vi "界面1-项目.vi"() -> ()   [LabVIEW 2013]
uses:
  GlobleVar/IndentLevel.vi
panel:
  out "Boolean":bool
  in  "<-硬件配置":bool
  in  "试验->":bool
  in  "实验结果汇总":string(tree)
  in  "项目管理":string(tree)
  in  "分析数据":bool
  in  "打印报告":bool
  in  "新建":bool
  in  "删除":bool
  in  "刷新":bool
  in  "重命名":bool
  in  "还原":bool
  in  "新建油动机":bool
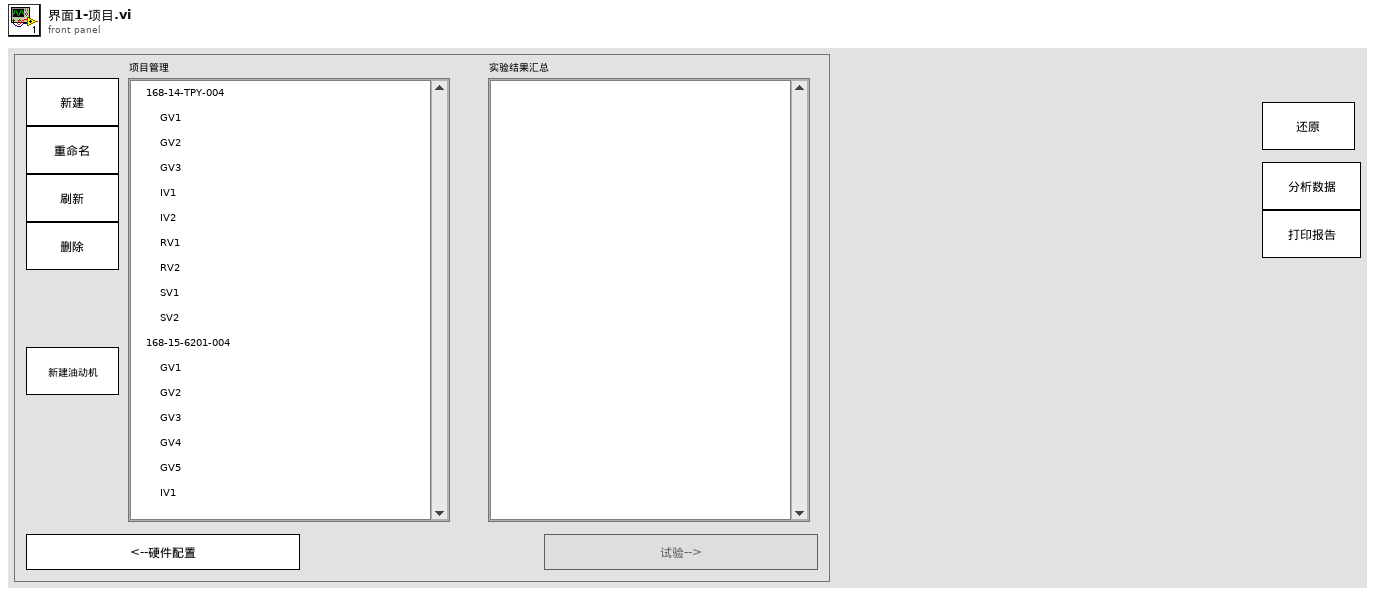
[diagram p1: front panel]
types:
  T1 = enum8{"Enabled", "Disabled", "Disabled and Grayed Out"}
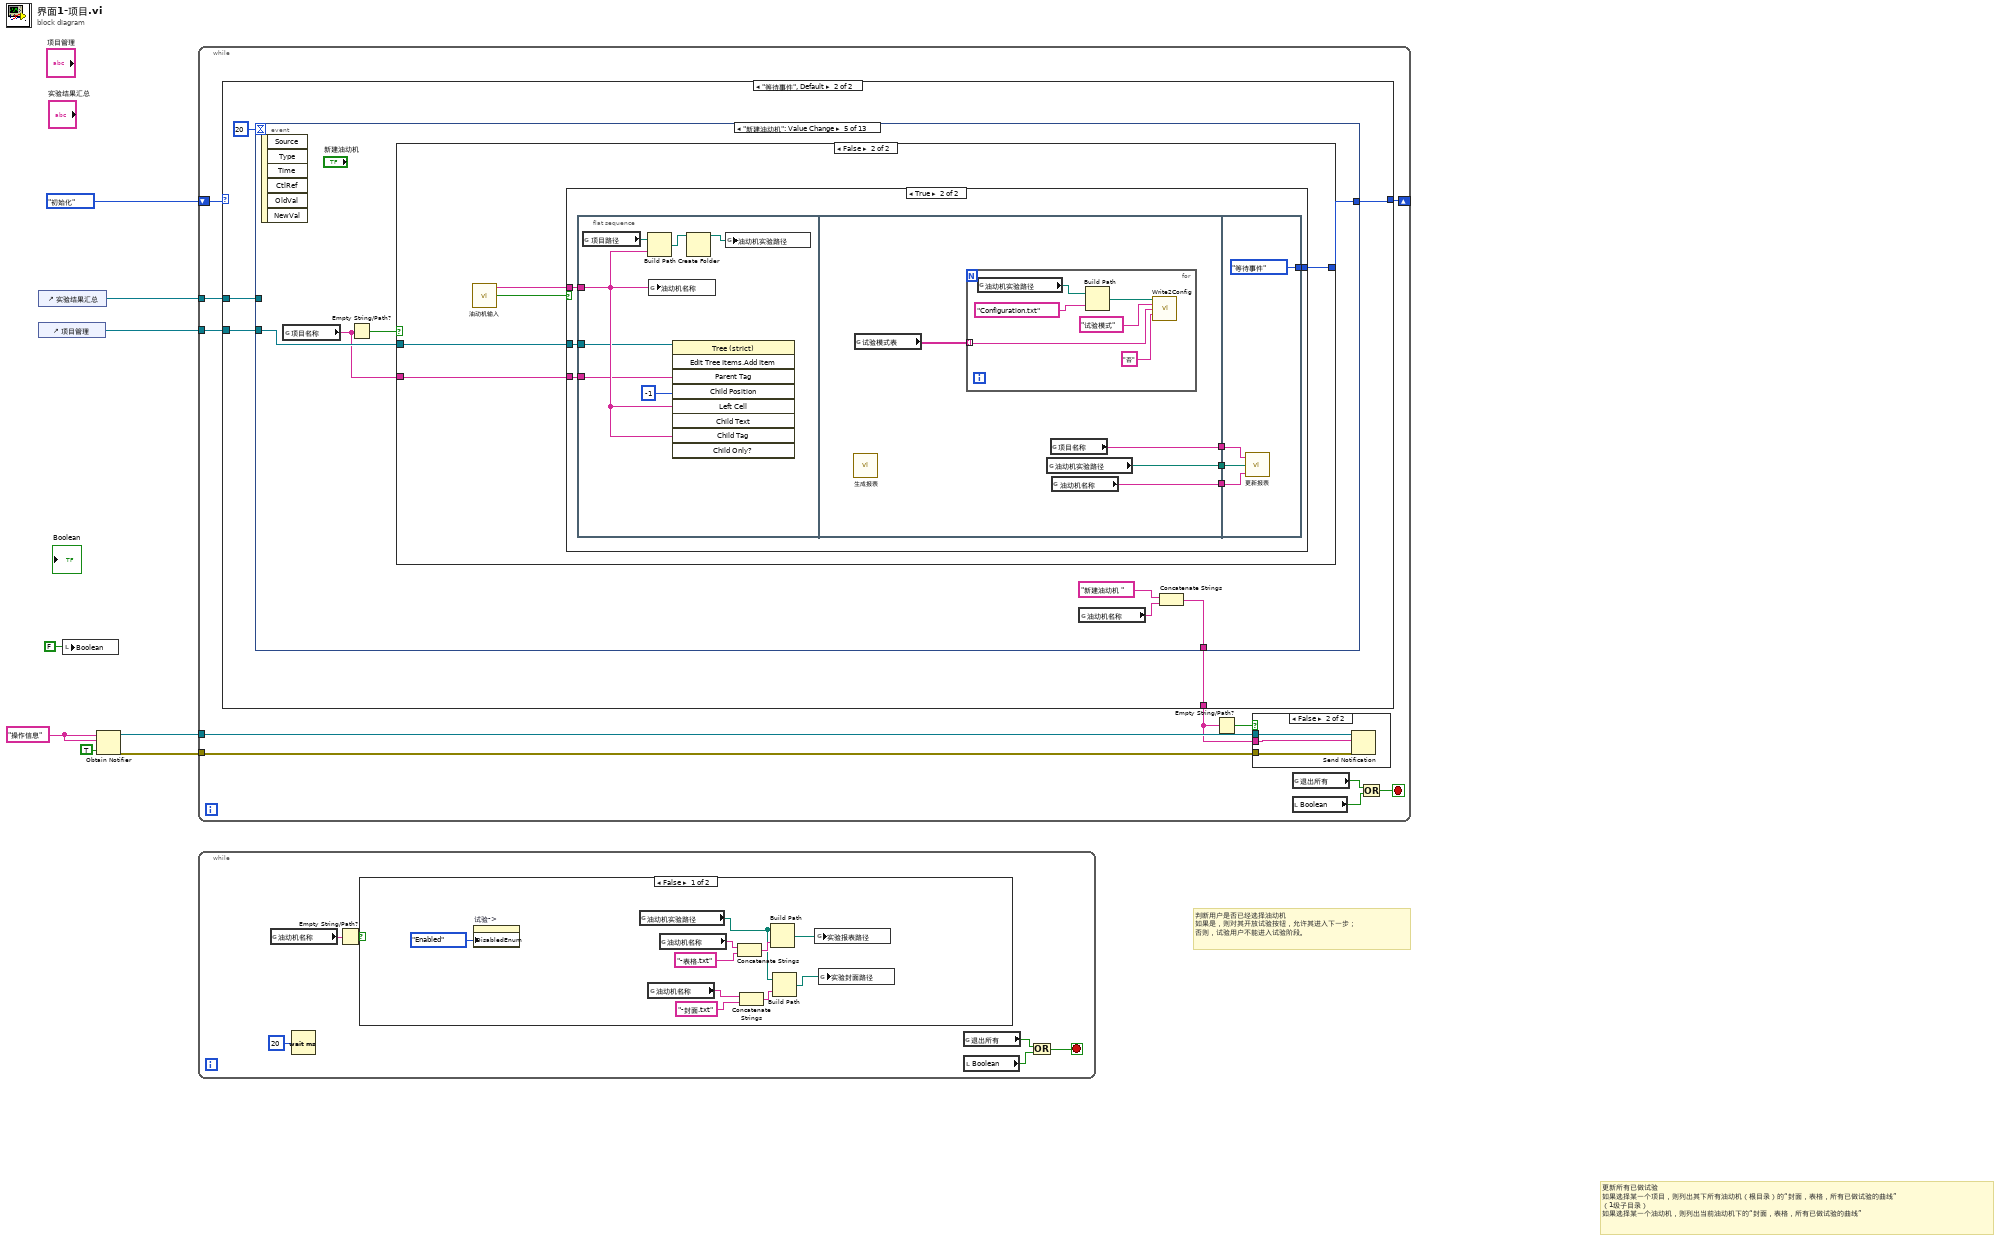
[diagram p0: block diagram]
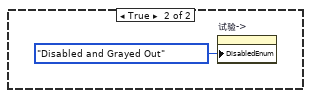
[diagram p2: hidden frame]
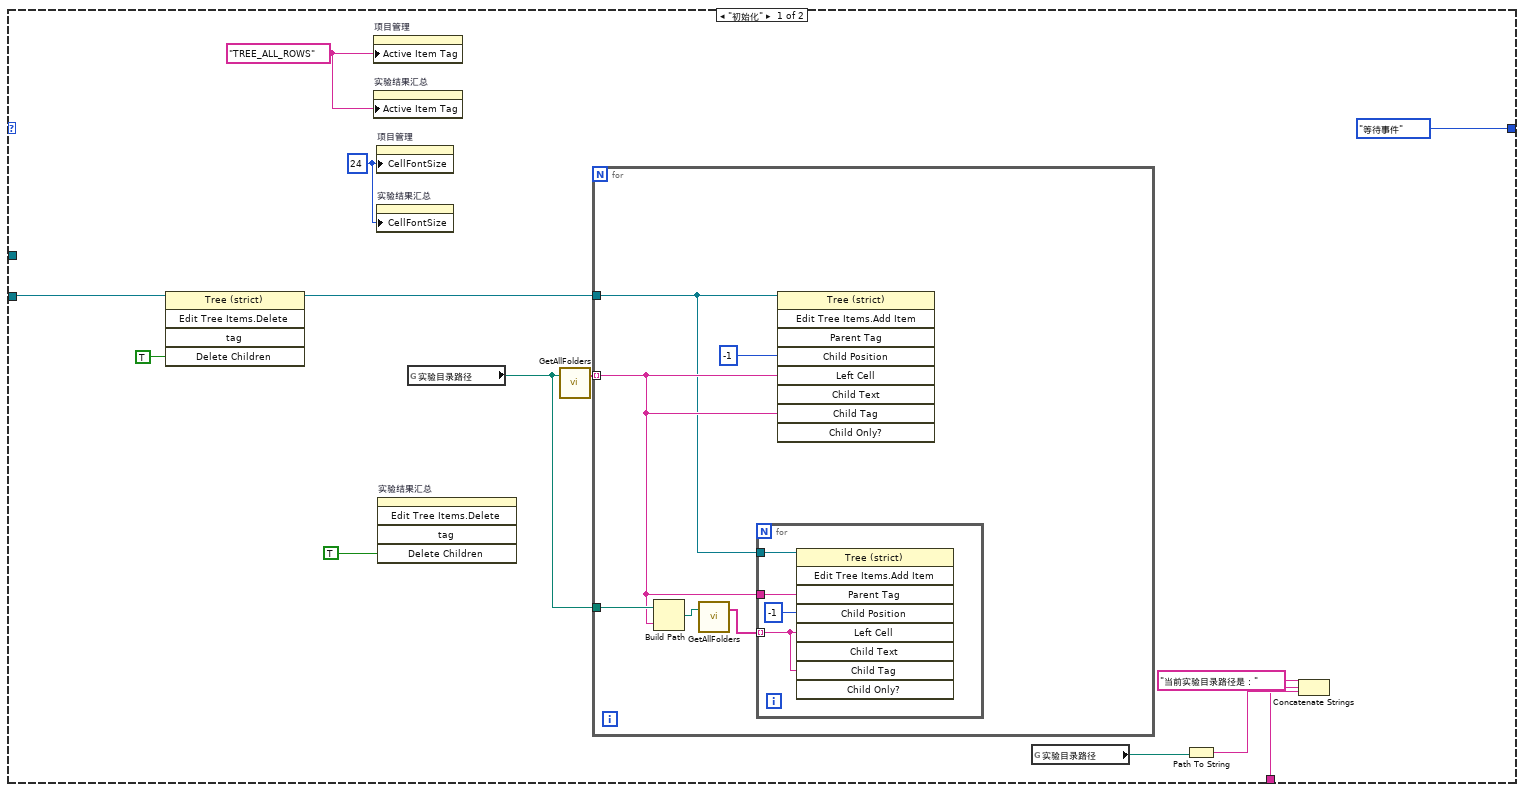
[diagram p4: hidden frame]
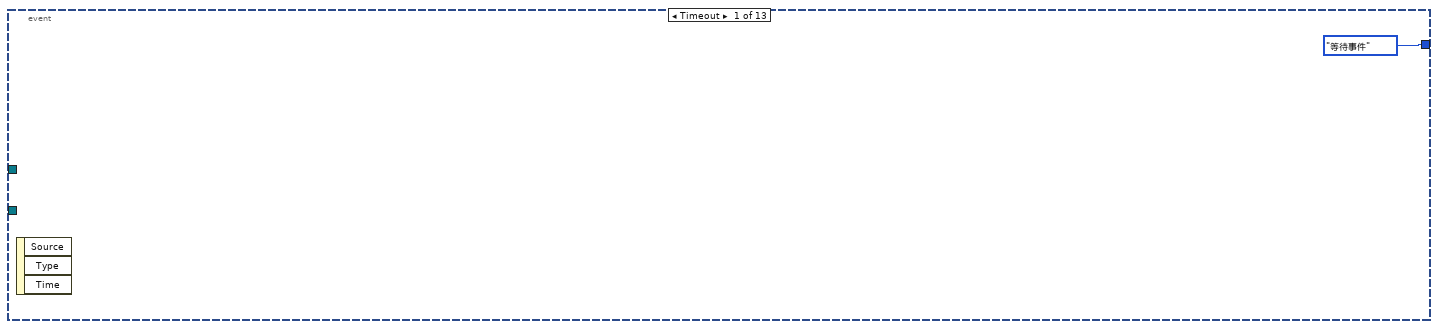
[diagram p5: hidden frame]
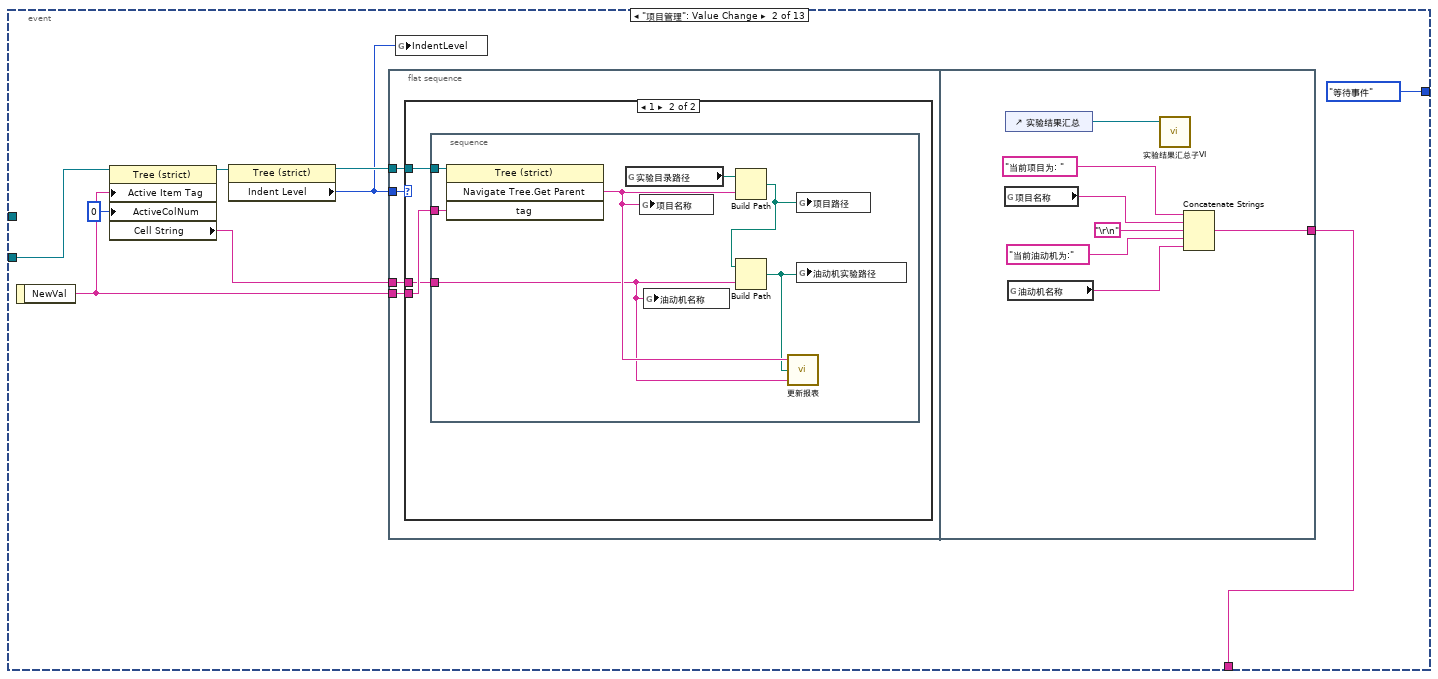
[diagram p6: hidden frame]
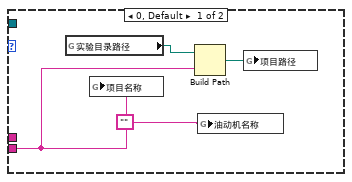
[diagram p7: hidden frame]
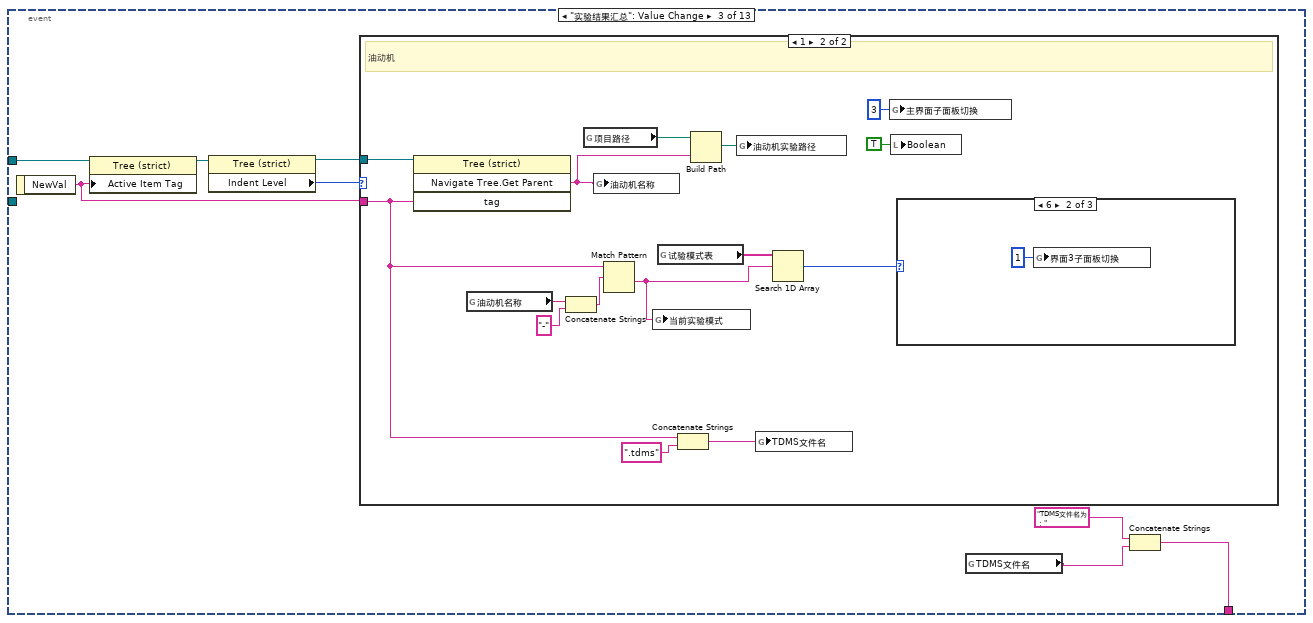
[diagram p8: hidden frame]
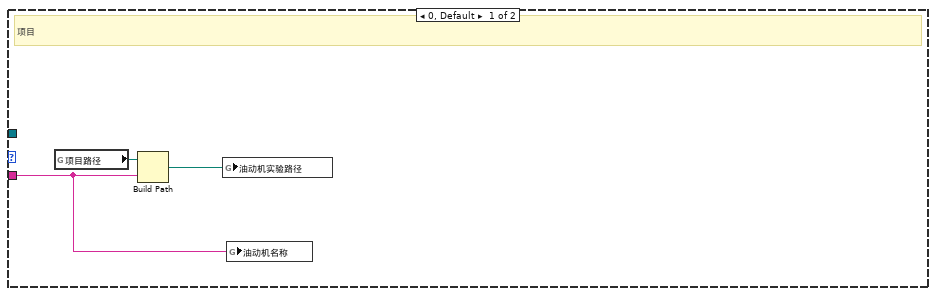
[diagram p9: hidden frame]
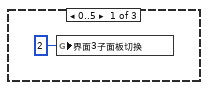
[diagram p10: hidden frame]
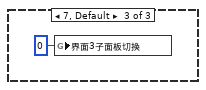
[diagram p11: hidden frame]
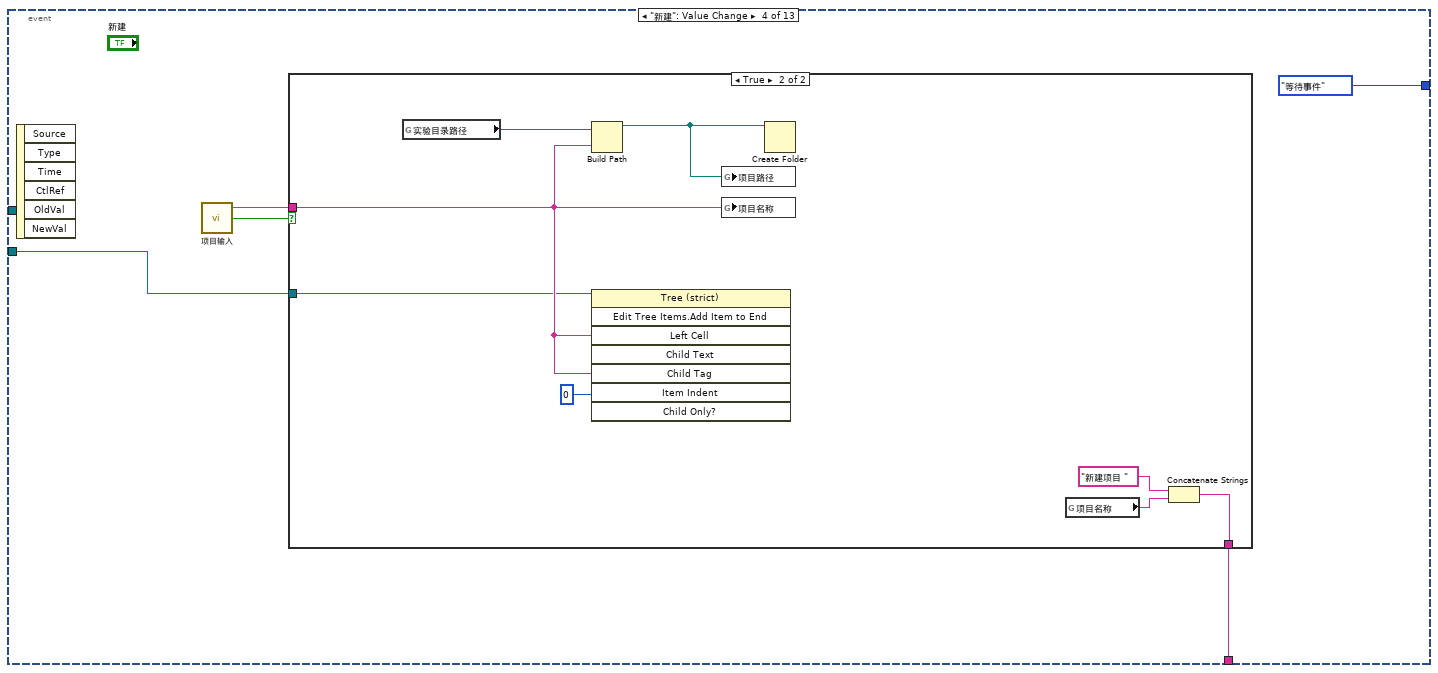
[diagram p12: hidden frame]
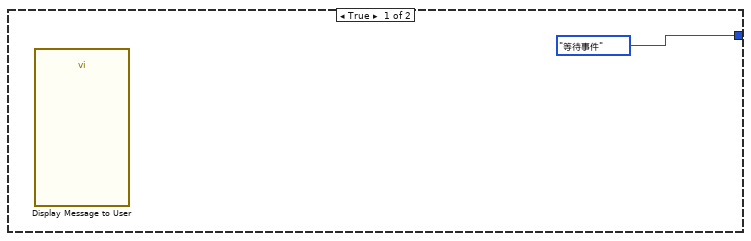
[diagram p14: hidden frame]
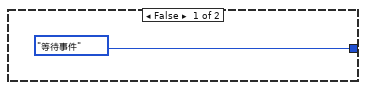
[diagram p15: hidden frame]
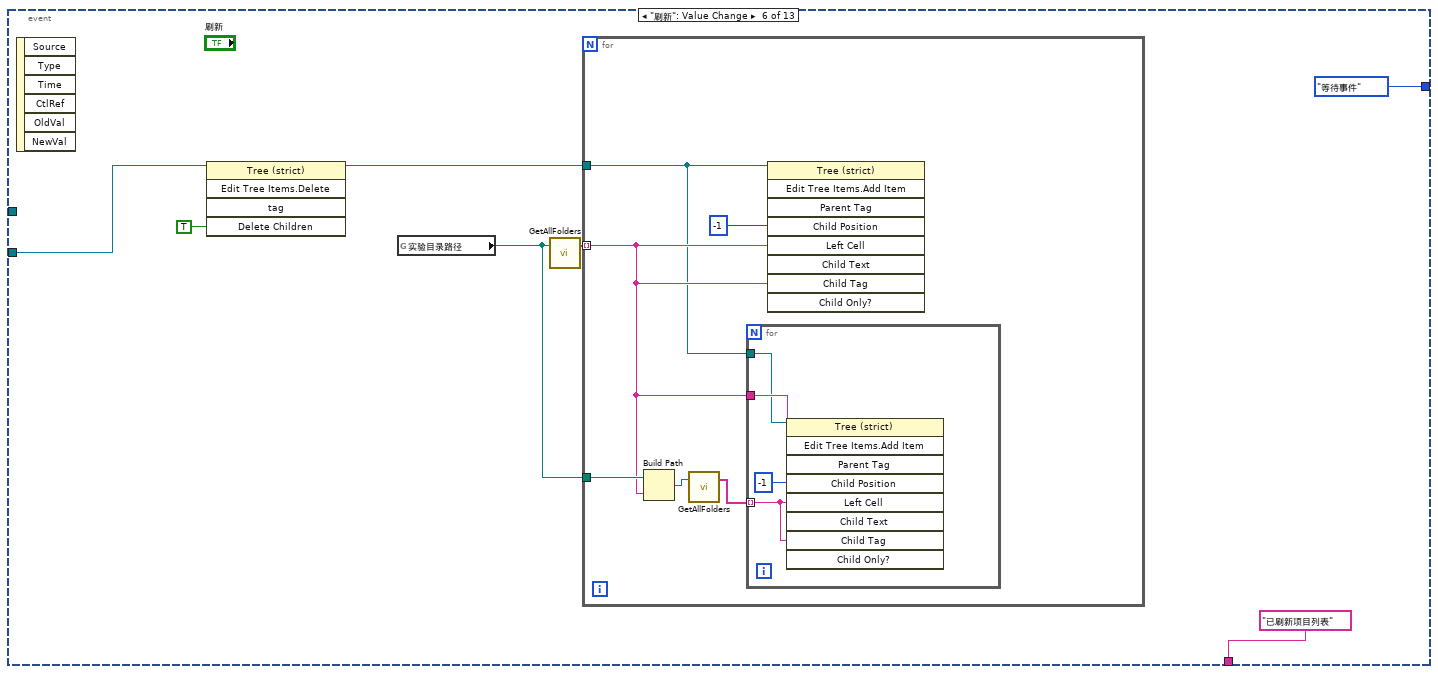
[diagram p16: hidden frame]
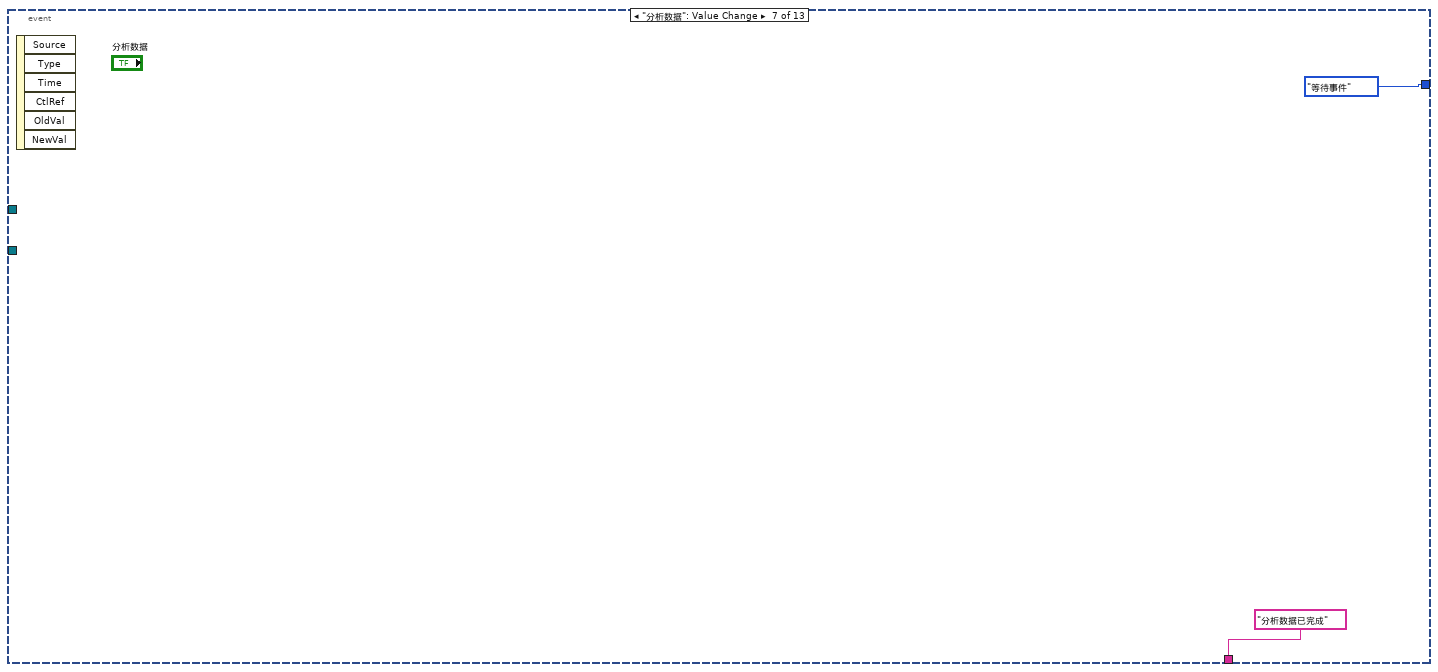
[diagram p17: hidden frame]
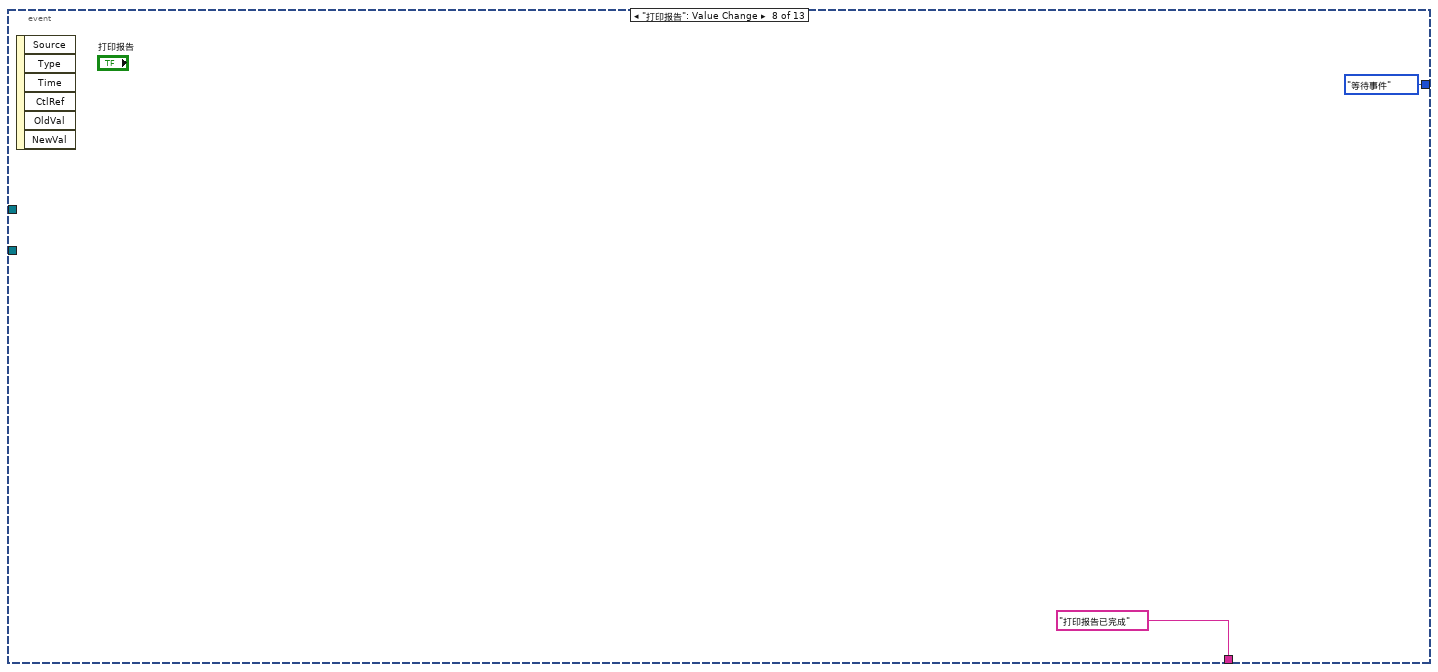
[diagram p18: hidden frame]
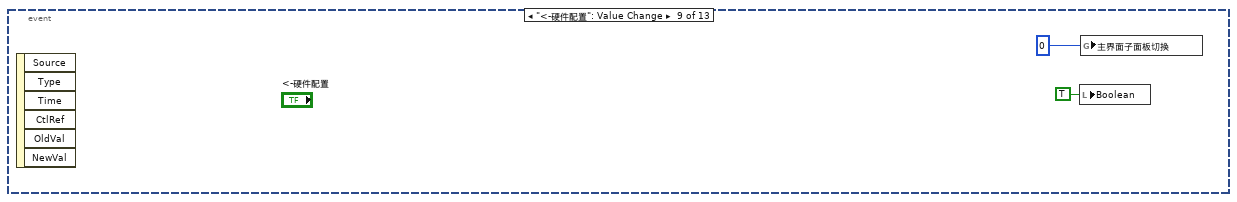
[diagram p19: hidden frame]
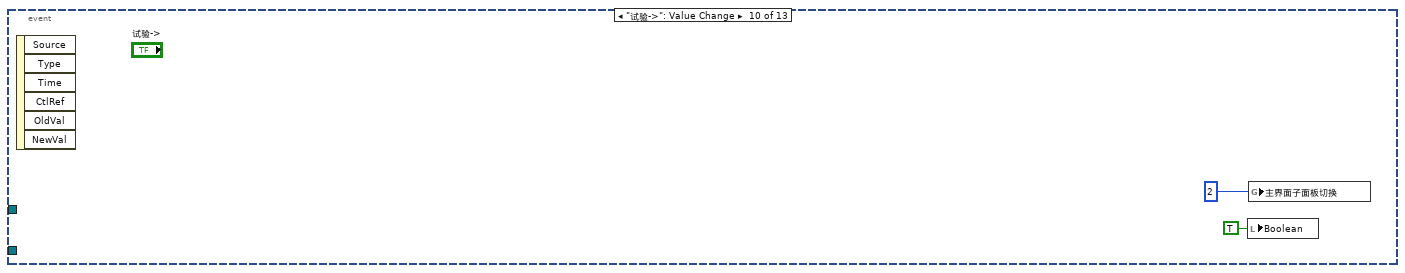
[diagram p20: hidden frame]
diagram:
  w7 = "操作信息"
  # "更新所有已做试验\n如果选择某一个项目，则列出其下所有油动机（根目录）的“封面，表格，所有已做试验的曲线”\n（1级子目录）\n如果选择某一个油动机，则列出当前油动机下的“封面，表格，所有已做试验的曲线”"
  # "判断用户是否已经选择油动机\n如果是，则对其开放试验按钮，允许其进入下一步；\n否则，试验用户不能进入试验阶段。"
  n1 = control-ref of="项目管理"() -> (w3:refnum<vi>)
  n2 = control-ref of="实验结果汇总"() -> (w1:refnum<vi>)
  n3 = local write "Boolean"(FALSE ("Boolean")) -> ()
  n4 = Obtain Notifier(name (unnamed)=w7, notification data type=w7, create if not found? (T)=TRUE) -> (notifier out=w6:refnum<notifier>, error out=w5:errorcluster)  [unwired: 1 in, 1 out]
  n5 = while {
    tunnel: w6 -> [w19]
    tunnel: w5 -> [w18]
    shift-right: [w15] -> _
    shift-left: enum16{"初始化", "等待事件", "退出"}."初始化" -> [w17]
    tunnel: w3 -> [w16]
    tunnel: w1 -> [w11]
    stop <- w12 stop-if-true
    n6 = case shown="\"等待事件\", Default" w17 {
      tunnel: w16 -> [w30 w50]
      tunnel: [w23 w49] -> w9
      tunnel: [enum16{"初始化", "等待事件", "退出"}."等待事件" w48] -> w15
      tunnel: w11 -> [_ w46]
      frame "初始化" {
        w34 = "TREE_ALL_ROWS" ("Active Item:Tag")
        w33 = u32 24 ("Active Cell:Cell Font:Size")
        n7 = invoke class="Tree (strict)" method="Edit Tree Items.Delete"(reference=w30, "Delete Children"=TRUE) -> (reference out=w27:refnum<vi>)  [unwired: 3 in, 4 out]
        n8 = property on="项目管理" class="Tree (strict)"("Active Item Tag"=w34) -> ()  [unwired: 2 in, 2 out]
        n9 = property on="实验结果汇总" class="Tree (strict)"("Active Item Tag"=w34) -> ()  [unwired: 2 in, 2 out]
        n10 = property on="项目管理" class="Tree (strict)"("CellFontSize"=w33) -> ()  [unwired: 2 in, 2 out]
        n11 = property on="实验结果汇总" class="Tree (strict)"("CellFontSize"=w33) -> ()  [unwired: 2 in, 2 out]
        n12 = invoke on="实验结果汇总" class="Tree (strict)" method="Edit Tree Items.Delete"("Delete Children"=TRUE ("Delete Children?")) -> ()  [unwired: 4 in, 5 out]
        n13 = global read "实验目录路径.vi" "实验目录路径"() -> (w28:path)
        n14 = call "GetAllFolders.vi"("FolderPath"=w28) -> ("Folders"=w29:string[])  [unwired: 1 in, 1 out]
        n15 = for {
          tunnel: w29 -> [w37] mode=indexing
          tunnel: w27 -> [w36]
          tunnel: w28 -> [w40]
          n16 = Build Path(base path=w40, name or relative path=w37) -> (appended path=w39:path)
          n17 = call "GetAllFolders.vi"("FolderPath"=w39) -> ("Folders"=w38:string[])  [unwired: 1 in, 1 out]
          n18 = for {
            tunnel: w38 -> [w45] mode=indexing
            tunnel: w37 -> [w44]
            tunnel: w36 -> [w42]
            n19 = invoke class="Tree (strict)" method="Edit Tree Items.Add Item"(reference=w42, "Parent Tag"=w44, "Child Position"=-1, "Left Cell"=w45, "Child Tag"=w45) -> ()  [unwired: 4 in, 9 out]
          }
          n20 = invoke class="Tree (strict)" method="Edit Tree Items.Add Item"(reference=w36, "Child Position"=-1, "Left Cell"=w37, "Child Tag"=w37) -> ()  [unwired: 5 in, 9 out]
        }
        n21 = global read "实验目录路径.vi" "实验目录路径"() -> (w26:path)
        n22 = Path To String(path=w26) -> (string=w24:string)
        n23 = Concatenate Strings("当前实验目录路径是：", w24) -> (w23:string)
      }
      frame "等待事件", Default {
        n24 = event shown="[4] \"新建油动机\": Value Change" {
          selector: _ -> [_ _ _ _ _ _ _ _ _ _ _ _ _]
          dyn-events: _ -> [_ _ _ _ _ _ _ _ _ _ _ _ _]
          timeout: 20 -> [_ _ _ _ _ _ _ _ _ _ _ _ _]
          tunnel: [enum16{"初始化", "等待事件", "退出"}."等待事件" enum16{"初始化", "等待事件", "退出"}."等待事件" _ enum16{"初始化", "等待事件", "退出"}."等待事件" w134 enum16{"初始化", "等待事件", "退出"}."等待事件" enum16{"初始化", "等待事件", "退出"}."等待事件" enum16{"初始化", "等待事件", "退出"}."等待事件" _ _ enum16{"初始化", "等待事件", "退出"}."初始化" enum16{"初始化", "等待事件", "退出"}."等待事件" enum16{"初始化", "等待事件", "退出"}."初始化"] -> w48
          tunnel: w50 -> [_ w57 _ w117 w132 w175 _ _ _ _ _ _ _]
          tunnel: [_ w55 w88 w115 w128 "已刷新项目列表" "分析数据已完成" "打印报告已完成" _ _ w197 _ w238] -> w49
          tunnel: w46 -> [_ _ w92 _ _ _ _ _ _ _ _ _ _]
          event Timeout {
            n25 = event-data() -> ()  [unwired: 1 in, 3 out]
          }
          event "项目管理": Value Change {
            n26 = event-data() -> ("NewVal"=w56:string)  [unwired: 1 in]
            n27 = property class="Tree (strict)"(reference=w57, "Active Item Tag"=w56, "ActiveColNum"=0 ("Active Cell:Active Column Number")) -> (reference out=w59:refnum<vi>, "Cell String"=w52:string)  [unwired: 1 in, 1 out]
            n28 = property class="Tree (strict)"(reference=w59) -> (reference out=w58:refnum<vi>, "Indent Level"=w54:i32)  [unwired: 1 in, 1 out]
            n29 = flat-sequence {
              tunnel: w54 -> [w64]
              tunnel: w58 -> [w63]
              tunnel: w56 -> [w62]
              tunnel: w52 -> [w61]
              tunnel: [w80] -> w55
              frame #0 {
                n30 = case shown="1" w64 {
                  tunnel: w62 -> [w65 w70]
                  tunnel: w63 -> [_ w71]
                  tunnel: w61 -> [_ w69]
                  frame 0, Default {
                    n31 = global read "实验目录路径.vi" "实验目录路径"() -> (w67:path)
                    n32 = global write "项目名称.vi" "项目名称"(w65) -> ()
                    n33 = Build Path(base path=w67, name or relative path=w65) -> (appended path=w66:path)
                    n34 = global write "油动机名称.vi" "油动机名称"("") -> ()
                    n35 = global write "项目路径.vi" "项目路径"(w66) -> ()
                  }
                  frame 1 {
                    n36 = stacked-sequence {
                      tunnel: w71 -> [w76]
                      tunnel: w70 -> [w75]
                      tunnel: w69 -> [w73]
                      frame #0 {
                        n37 = invoke class="Tree (strict)" method="Navigate Tree.Get Parent"(reference=w76, "tag"=w75) -> ("Navigate Tree:Get Parent"=w74:string)  [unwired: 2 in, 3 out]
                        n38 = global read "实验目录路径.vi" "实验目录路径"() -> (w78:path)
                        n39 = global write "项目名称.vi" "项目名称"(w74) -> ()
                        n40 = global write "油动机名称.vi" "油动机名称"(w73) -> ()
                        n41 = Build Path(base path=w78, name or relative path=w74) -> (appended path=w77:path)
                        n42 = Build Path(base path=w77, name or relative path=w73) -> (appended path=w72:path)
                        n43 = call "更新报表.vi"("油动机名称"=w73, "油动机试验路径"=w72, "项目名称"=w74) -> ()  [unwired: 3 in]
                        n44 = global write "项目路径.vi" "项目路径"(w77) -> ()
                        n45 = global write "油动机实验路径.vi" "油动机实验路径"(w72) -> ()
                      }
                    }
                  }
                }
              }
              frame #1 {
                n46 = global read "项目名称.vi" "项目名称"() -> (w83:string)
                n47 = control-ref of="实验结果汇总"() -> (w79:refnum<vi>)
                n48 = global read "油动机名称.vi" "油动机名称"() -> (w85:string)
                n49 = call "实验结果汇总子VI.vi"("reference in"=w79) -> ()  [unwired: 5 in]
                n50 = Concatenate Strings("当前项目为: ", w83, "\r\n", "当前油动机为:", w85) -> (w80:string)
              }
            }
            n51 = global write "IndentLevel.vi" "IndentLevel"(w54) -> ()
          }
          event "实验结果汇总": Value Change {
            n52 = event-data() -> ("NewVal"=w87:string)  [unwired: 1 in]
            n53 = property class="Tree (strict)"(reference=w92, "Active Item Tag"=w87) -> (reference out=w93:refnum<vi>)  [unwired: 1 in, 1 out]
            n54 = property class="Tree (strict)"(reference=w93) -> (reference out=w91:refnum<vi>, "Indent Level"=w90:i32)  [unwired: 1 in, 1 out]
            n55 = case shown="1" w90 {
              tunnel: w91 -> [_ w111]
              tunnel: w87 -> [w94 w98]
              frame 0, Default {
                # "项目"
                n56 = global read "项目路径.vi" "项目路径"() -> (w96:path)
                n57 = Build Path(base path=w96, name or relative path=w94) -> (appended path=w95:path)
                n58 = global write "油动机实验路径.vi" "油动机实验路径"(w95) -> ()
                n59 = global write "油动机名称.vi" "油动机名称"(w94) -> ()
              }
              frame 1 {
                # "油动机"
                n60 = invoke class="Tree (strict)" method="Navigate Tree.Get Parent"(reference=w111, "tag"=w98) -> ("Navigate Tree:Get Parent"=w110:string)  [unwired: 2 in, 3 out]
                n61 = global read "油动机名称.vi" "油动机名称"() -> (w105:string)
                n62 = Concatenate Strings(w105, "-") -> (w99:string)
                n63 = global read "项目路径.vi" "项目路径"() -> (w109:path)
                n64 = global write "油动机名称.vi" "油动机名称"(w110) -> ()
                n65 = Match Pattern(string=w98, regular expression=w99) -> (after substring=w103:string)  [unwired: 1 in, 3 out]
                n66 = global write "当前实验模式.vi" "当前实验模式"(w103) -> ()
                n67 = global read "试验模式表.vi" "试验模式表"() -> (w102:string[])
                n68 = Concatenate Strings(w98, ".tdms") -> (w100:string)
                n69 = Build Path(base path=w109, name or relative path=w110) -> (appended path=w108:path)
                n70 = global write "油动机实验路径.vi" "油动机实验路径"(w108) -> ()
                n71 = global write "TDMS文件名.vi" "TDMS文件名"(w100) -> ()
                n72 = Search 1D Array(1D array=w102, element=w103) -> (index of element=w101:i32)  [unwired: 1 in]
                n73 = global write "主界面子面板切换.vi" "主界面子面板切换"(3 ("主界面子面板切换")) -> ()
                n74 = local write "Boolean"(TRUE ("Boolean")) -> ()
                n75 = case shown="6" w101 {
                  frame 0..5 {
                    n76 = global write "界面3子面板切换.vi" "界面3子面板切换"(2 ("界面3子面板切换")) -> ()
                  }
                  frame 6 {
                    n77 = global write "界面3子面板切换.vi" "界面3子面板切换"(1 ("界面3子面板切换")) -> ()
                  }
                  frame 7, Default {
                    n78 = global write "界面3子面板切换.vi" "界面3子面板切换"(0 ("界面3子面板切换")) -> ()
                  }
                }
              }
            }
            n79 = global read "TDMS文件名.vi" "TDMS文件名"() -> (w86:string)
            n80 = Concatenate Strings("TDMS文件名为：", w86) -> (w88:string)
          }
          event "新建": Value Change {
            n81 = event-data() -> ()  [unwired: 1 in, 6 out]
            n82 = call "项目输入.vi"() -> ("输入有效"=w116:bool, "项目名称"=w118:string)  [unwired: 4 in]
            n83 = case shown="True" w116 {
              tunnel: w118 -> [_ w124]
              tunnel: w117 -> [_ w123]
              tunnel: [_ w120] -> w115
              frame False {
              }
              frame True {
                n84 = global read "实验目录路径.vi" "实验目录路径"() -> (w125:path)
                n85 = Build Path(base path=w125, name or relative path=w124) -> (appended path=w126:path)
                n86 = invoke class="Tree (strict)" method="Edit Tree Items.Add Item to End"(reference=w123, "Left Cell"=w124, "Child Tag"=w124, "Item Indent"=0) -> ()  [unwired: 4 in, 8 out]
                n87 = global write "项目路径.vi" "项目路径"(w126) -> ()
                n88 = global write "项目名称.vi" "项目名称"(w124) -> ()
                n89 = Create Folder(path (use dialog)=w126) -> ()  [unwired: 2 in, 3 out]
                n90 = global read "项目名称.vi" "项目名称"() -> (w122:string)
                n91 = Concatenate Strings("新建项目 ", w122) -> (w120:string)
              }
            }
          }
          event "新建油动机": Value Change {
            n92 = event-data() -> ()  [unwired: 1 in, 6 out]
            n93 = global read "项目名称.vi" "项目名称"() -> (w131:string)
            n94 = Empty String/Path?(string/path=w131) -> (empty?=w133:bool)
            n95 = case shown="False" w133 {
              tunnel: [enum16{"初始化", "等待事件", "退出"}."等待事件" w140] -> w134
              tunnel: w132 -> [_ w139]
              tunnel: w131 -> [_ w138]
              frame True {
                n96 = call "Display Message to User"() -> ()  [unwired: 10 in, 2 out]
              }
              frame False {
                n97 = call "油动机输入.vi"() -> ("输入有效"=w137:bool, "油动机名称"=w136:string)  [unwired: 4 in]
                n98 = case shown="True" w137 {
                  tunnel: w136 -> [_ w148]
                  tunnel: [enum16{"初始化", "等待事件", "退出"}."等待事件" w147] -> w140
                  tunnel: w139 -> [_ w146]
                  tunnel: w138 -> [_ w145]
                  frame False {
                  }
                  frame True {
                    n99 = flat-sequence {
                      tunnel: w148 -> [w151]
                      tunnel: w146 -> [w150]
                      tunnel: w145 -> [w149]
                      tunnel: [w158] -> w144
                      tunnel: [w157] -> w143
                      tunnel: [w156] -> w142
                      tunnel: [enum16{"初始化", "等待事件", "退出"}."等待事件"] -> w147
                      tunnel: w144 -> [w168]
                      tunnel: w143 -> [w167]
                      tunnel: w142 -> [w166]
                      frame #0 {
                        n100 = global read "项目路径.vi" "项目路径"() -> (w155:path)
                        n101 = Build Path(base path=w155, name or relative path=w151) -> (appended path=w154:path)
                        n102 = global write "油动机名称.vi" "油动机名称"(w151) -> ()
                        n103 = invoke class="Tree (strict)" method="Edit Tree Items.Add Item"(reference=w150, "Parent Tag"=w149, "Child Position"=-1, "Left Cell"=w151, "Child Tag"=w151) -> ()  [unwired: 4 in, 9 out]
                        n104 = Create Folder(path (use dialog)=w154) -> (created path=w153:path)  [unwired: 2 in, 2 out]
                        n105 = global write "油动机实验路径.vi" "油动机实验路径"(w153) -> ()
                      }
                      frame #1 {
                        n106 = call "生成报表.vi"() -> ()  [unwired: 6 in]
                        n107 = global read "试验模式表.vi" "试验模式表"() -> (w159:string[])
                        n108 = for {
                          tunnel: w159 -> [w161] mode=indexing
                          n109 = global read "油动机实验路径.vi" "油动机实验路径"() -> (w165:path)
                          n110 = Build Path(base path=w165, name or relative path="Configuration.txt") -> (appended path=w163:path)
                          n111 = call "Write2Config.vi"("Path"=w163, "Section"="试验模式", "Key"=w161, "Value"="否") -> ()  [unwired: 11 in, 1 out]
                        }
                        n112 = global read "油动机实验路径.vi" "油动机实验路径"() -> (w158:path)
                        n113 = global read "项目名称.vi" "项目名称"() -> (w156:string)
                        n114 = global read "油动机名称.vi" "油动机名称"() -> (w157:string)
                      }
                      frame #2 {
                        n115 = call "更新报表.vi"("油动机名称"=w167, "油动机试验路径"=w168, "项目名称"=w166) -> ()  [unwired: 3 in]
                      }
                    }
                  }
                }
              }
            }
            n116 = global read "油动机名称.vi" "油动机名称"() -> (w129:string)
            n117 = Concatenate Strings("新建油动机 ", w129) -> (w128:string)
          }
          event "刷新": Value Change {
            n118 = event-data() -> ()  [unwired: 1 in, 6 out]
            n119 = invoke class="Tree (strict)" method="Edit Tree Items.Delete"(reference=w175, "Delete Children"=TRUE) -> (reference out=w170:refnum<vi>)  [unwired: 3 in, 4 out]
            n120 = global read "实验目录路径.vi" "实验目录路径"() -> (w171:path)
            n121 = call "GetAllFolders.vi"("FolderPath"=w171) -> ("Folders"=w172:string[])  [unwired: 1 in, 1 out]
            n122 = for {
              tunnel: w172 -> [w178] mode=indexing
              tunnel: w170 -> [w177]
              tunnel: w171 -> [w181]
              n123 = Build Path(base path=w181, name or relative path=w178) -> (appended path=w180:path)
              n124 = call "GetAllFolders.vi"("FolderPath"=w180) -> ("Folders"=w179:string[])  [unwired: 1 in, 1 out]
              n125 = for {
                tunnel: w179 -> [w186] mode=indexing
                tunnel: w178 -> [w185]
                tunnel: w177 -> [w183]
                n126 = invoke class="Tree (strict)" method="Edit Tree Items.Add Item"(reference=w183, "Parent Tag"=w185, "Child Position"=-1, "Left Cell"=w186, "Child Tag"=w186) -> ()  [unwired: 4 in, 9 out]
              }
              n127 = invoke class="Tree (strict)" method="Edit Tree Items.Add Item"(reference=w177, "Child Position"=-1, "Left Cell"=w178, "Child Tag"=w178) -> ()  [unwired: 5 in, 9 out]
            }
          }
          event "分析数据": Value Change {
            n128 = event-data() -> ()  [unwired: 1 in, 6 out]
          }
          event "打印报告": Value Change {
            n129 = event-data() -> ()  [unwired: 1 in, 6 out]
          }
          event "<-硬件配置": Value Change {
            n130 = event-data() -> ()  [unwired: 1 in, 6 out]
            n131 = local write "Boolean"(TRUE ("Boolean")) -> ()
            n132 = global write "主界面子面板切换.vi" "主界面子面板切换"(0) -> ()
          }
          event "试验->": Value Change {
            n133 = event-data() -> ()  [unwired: 1 in, 6 out]
            n134 = local write "Boolean"(TRUE ("Boolean")) -> ()
            n135 = global write "主界面子面板切换.vi" "主界面子面板切换"(2) -> ()
          }
          event "删除": Value Change {
            n136 = event-data() -> ()  [unwired: 1 in, 6 out]
            n137 = global read "油动机名称.vi" "油动机名称"() -> (w195:string)
            n138 = Empty String/Path?(string/path=w195) -> (empty?=w198:bool)
            n139 = case shown="True" w198 {
              tunnel: [w200 w217] -> w197
              tunnel: w195 -> [w199 _]
              frame False {
                # "删除油动机文件夹下所有文件"
                n140 = Concatenate Strings("删除后不可恢复，确认删除油动机" ("message"), w199) -> (w204:string)
                n141 = Two Button Dialog(message=w204, 1:"取消" ("F button name (\"Cancel\")"), 2:"确认" ("T button name (\"OK\")")) -> (T button?=w201:bool)
                n142 = case shown="True" w201 {
                  tunnel: ["油动机删除操作已取消" "油动机已删除"] -> w200
                  frame False {
                  }
                  frame True {
                    n143 = global read "油动机实验路径.vi" "油动机实验路径"() -> (w208:path)
                    n144 = Path To String(path=w208) -> (string=w213:string)
                    n145 = Concatenate Strings("cmd /c ", "rd /s /q ", "\"", w213, "\"") -> (w211:string)
                    n146 = call <vilib>:"System Exec.vi"("run minimized? (F)"=FALSE, "command line"=w211) -> ()  [unwired: 6 in, 4 out]
                  }
                }
              }
              frame True {
                n147 = global read "项目名称.vi" "项目名称"() -> (w216:string)
                n148 = Empty String/Path?(string/path=w216) -> (empty?=w218:bool)
                n149 = case shown="False" w218 {
                  tunnel: [w219 _] -> w217
                  tunnel: w216 -> [w223 _]
                  frame False {
                    # "删除整个项目"
                    n150 = Concatenate Strings("删除后不可恢复，确认删除项目" ("message"), w223) -> (w222:string)
                    n151 = Two Button Dialog(message=w222, 1:"取消" ("F button name (\"Cancel\")"), 2:"确认" ("T button name (\"OK\")")) -> (T button?=w225:bool)
                    n152 = case shown="True" w225 {
                      tunnel: ["项目删除操作已取消" "项目已删除"] -> w219
                      frame False {
                      }
                      frame True {
                        n153 = global read "项目路径.vi" "项目路径"() -> (w235:path)
                        n154 = Path To String(path=w235) -> (string=w232:string)
                        n155 = Concatenate Strings("cmd /c ", "rd /s /q ", "\"", w232, "\"") -> (w230:string)
                        n156 = call <vilib>:"System Exec.vi"("run minimized? (F)"=FALSE, "command line"=w230) -> ()  [unwired: 6 in, 4 out]
                      }
                    }
                  }
                  frame True {
                  }
                }
              }
            }
          }
          event "还原": Value Change {
            n157 = event-data() -> ()  [unwired: 1 in, 6 out]
          }
          event "重命名": Value Change {
            n158 = event-data() -> ()  [unwired: 1 in, 6 out]
            n159 = global read "油动机名称.vi" "油动机名称"() -> (w239:string)
            n160 = Empty String/Path?(string/path=w239) -> (empty?=w240:bool)
            n161 = case shown="False" w240 {
              tunnel: [w241 w268] -> w238
              frame False {
                # "重命名油动机"
                n162 = call "油动机输入.vi"() -> ("输入有效"=w242:bool, "油动机名称"=w243:string)  [unwired: 4 in]
                n163 = case shown="True" w242 {
                  tunnel: ["油动机重命名操作已取消" "油动机已重命名"] -> w241
                  tunnel: w243 -> [_ w248]
                  frame False {
                  }
                  frame True {
                    n164 = flat-sequence {
                      tunnel: w248 -> [w250]
                      tunnel: [w254] -> w247
                      tunnel: [w250] -> w246
                      tunnel: w247 -> [w265]
                      tunnel: w246 -> [w263]
                      tunnel: [w263] -> w245
                      tunnel: w245 -> [w266]
                      frame #0 {
                        w253 = "\""
                        n165 = global read "项目路径.vi" "项目路径"() -> (w256:path)
                        n166 = global read "油动机实验路径.vi" "油动机实验路径"() -> (w255:path)
                        n167 = Build Path(base path=w256, name or relative path=w250) -> (appended path=w254:path)
                        n168 = Path To String(path=w254) -> (string=w252:string)
                        n169 = Path To String(path=w255) -> (string=w260:string)
                        n170 = Concatenate Strings("cmd /c ", "move ", "\"", w260, w253, " " ("string"), w253, w252, w253) -> (w259:string)
                        n171 = call <vilib>:"System Exec.vi"("run minimized? (F)"=FALSE, "command line"=w259) -> ()  [unwired: 6 in, 4 out]
                      }
                      frame #1 {
                        n172 = global read "油动机名称.vi" "油动机名称"() -> (w264:string)
                        n173 = global write "油动机实验路径.vi" "油动机实验路径"(w265) -> ()
                        n174 = call "RenameFiles.vi"("新油动机名称"=w263, "旧油动机名称"=w264, "Path"=w265) -> ()  [unwired: 3 in]
                      }
                      frame #2 {
                        n175 = global write "油动机名称.vi" "油动机名称"(w266) -> ()
                      }
                    }
                  }
                }
              }
              frame True {
                n176 = global read "项目名称.vi" "项目名称"() -> (w267:string)
                n177 = Empty String/Path?(string/path=w267) -> (empty?=w269:bool)
                n178 = case shown="False" w269 {
                  tunnel: [w272 _] -> w268
                  frame False {
                    # "重命名项目"
                    n179 = call "项目输入.vi"() -> ("输入有效"=w271:bool, "项目名称"=w270:string)  [unwired: 4 in]
                    n180 = case shown="True" w271 {
                      tunnel: ["项目重命名操作已取消" w274] -> w272
                      tunnel: w270 -> [_ w279]
                      frame False {
                      }
                      frame True {
                        n181 = flat-sequence {
                          tunnel: w279 -> [w284]
                          tunnel: [w283] -> w278
                          tunnel: w278 -> [w293]
                          tunnel: [w293] -> w277
                          frame #0 {
                            w281 = "\""
                            n182 = global read "实验目录路径.vi" "实验目录路径"() -> (w285:path)
                            n183 = global write "项目名称.vi" "项目名称"(w284) -> ()
                            n184 = global read "项目路径.vi" "项目路径"() -> (w292:path)
                            n185 = Build Path(base path=w285, name or relative path=w284) -> (appended path=w283:path)
                            n186 = Path To String(path=w283) -> (string=w282:string)
                            n187 = Path To String(path=w292) -> (string=w289:string)
                            n188 = Concatenate Strings("cmd /c ", "move ", "\"", w289, w281, " " ("string"), w281, w282, w281) -> (w288:string)
                            n189 = call <vilib>:"System Exec.vi"("run minimized? (F)"=FALSE, "command line"=w288) -> ()  [unwired: 6 in, 4 out]
                          }
                          frame #1 {
                            n190 = global write "项目路径.vi" "项目路径"(w293) -> ()
                          }
                        }
                        n191 = Path To String(path=w277) -> (string=w275:string)
                        n192 = Concatenate Strings("项目已重命名，新的项目路径为：\n", w275) -> (w274:string)
                      }
                    }
                  }
                  frame True {
                  }
                }
              }
            }
          }
        }
      }
    }
    n193 = Empty String/Path?(string/path=w9) -> (empty?=w10:bool)
    n194 = case shown="False" w10 {
      tunnel: w19 -> [_ w22]
      tunnel: w18 -> [_ w21]
      tunnel: w9 -> [_ w20]
      frame True {
      }
      frame False {
        n195 = Send Notification(notification=w20, notifier=w22, error in (no error)=w21) -> ()  [unwired: 2 out]
      }
    }
    n196 = global read "退出所有.vi" "退出所有"() -> (w14:bool)
    n197 = local read "Boolean"() -> (w13:bool)
    n198 = Or(x=w14, y=w13) -> (x .or. y?=w12:bool)
  }
  n199 = while {
    stop <- w294 stop-if-true
    n200 = global read "油动机名称.vi" "油动机名称"() -> (w299:string)
    n201 = Wait (ms)(milliseconds to wait=u32 20) -> ()  [unwired: 1 out]
    n202 = Empty String/Path?(string/path=w299) -> (empty?=w298:bool)
    n203 = case shown="False" w298 {
      frame False {
        n204 = property on="试验->" class="Bool"("DisabledEnum"=T1."Enabled" ("Disabled")) -> ()  [unwired: 2 in, 2 out]
        n205 = global read "油动机实验路径.vi" "油动机实验路径"() -> (w300:path)
        n206 = global read "油动机名称.vi" "油动机名称"() -> (w301:string)
        n207 = global read "油动机名称.vi" "油动机名称"() -> (w306:string)
        n208 = Concatenate Strings(w306, "-表格.txt") -> (w307:string)
        n209 = Concatenate Strings(w301, "-封面.txt") -> (w304:string)
        n210 = Build Path(base path=w300, name or relative path=w307) -> (appended path=w308:path)
        n211 = Build Path(base path=w300, name or relative path=w304) -> (appended path=w303:path)
        n212 = global write "实验报表路径.vi" "实验报表路径"(w308) -> ()
        n213 = global write "实验封面路径.vi" "实验封面路径"(w303) -> ()
      }
      frame True {
        n214 = property on="试验->" class="Bool"("DisabledEnum"=T1."Disabled and Grayed Out" ("Disabled")) -> ()  [unwired: 2 in, 2 out]
      }
    }
    n215 = global read "退出所有.vi" "退出所有"() -> (w296:bool)
    n216 = local read "Boolean"() -> (w295:bool)
    n217 = Or(x=w296, y=w295) -> (x .or. y?=w294:bool)
  }
